vi "Rectify Image (ARGB).vi"(5 "Crop to Valid Pixels? (Default: True)":bool=TRUE, 7 "Use Fixed Point Remapping (Default: False)":bool, 8 "error in (no error)":errorcluster, 9 "ARGB Image Destination":T1, 10 "ARGB Image Source":T1, 11 "ImageRectifier":refnum<class "ImageRectifier.lvclass">) -> (0 "error out":errorcluster, 2 "ARGB Image Destination (duplicate)":T1, 3 "ImageRectifier (Duplicate)":refnum<class "ImageRectifier.lvclass">)   [LabVIEW 2020, in "image.lvlib" / "ImageRectifier.lvclass"]
uses:
  ImageRectifier.lvclass
  ARGB Image.ctl
  ImageRectifier.lvclass/ImageRectifier.ctl
  ccc224f2-fea8-4097-85c8-c2b3fe04188f.vi
  common/Module Path.vi
  <vilib>/Utility/error.llb/Error Cluster From Error Code.vi
  image.lvlib
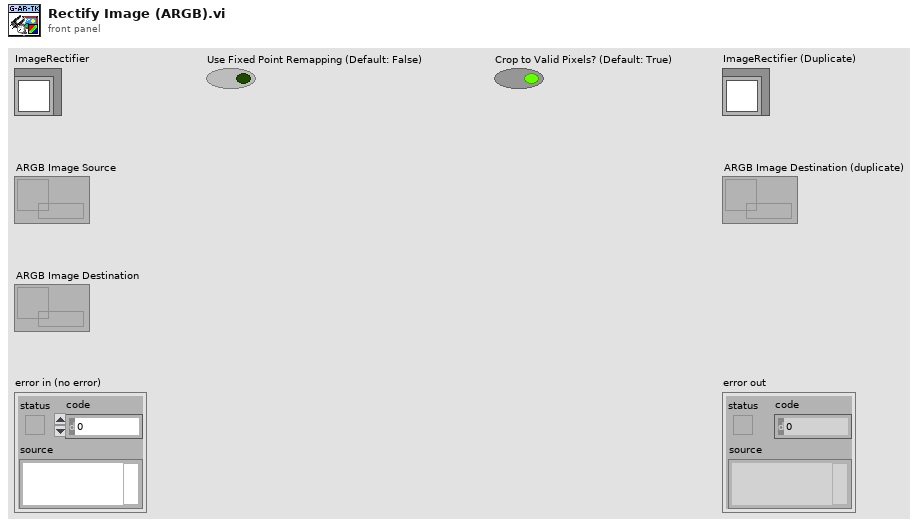
[diagram p1: front panel]
types:
  T1 = typedef "image.lvlib/ARGB Image.ctl" = refnum<data-value>
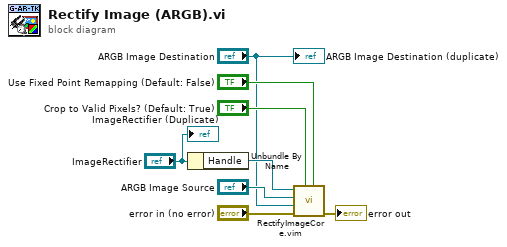
[diagram p0: block diagram]
diagram:
  n1 = Unbundle By Name("ImageRectifier") -> ("Handle"=w7:refnum<data-value>)
  n2 = call "RectifyImageCore.vim"("Use Fixed Point remapping"="Use Fixed Point Remapping (Default: False)", "Crop to Valid"="Crop to Valid Pixels? (Default: True)", "error in (no error)"="error in (no error)", "Destination Image"="ARGB Image Destination", "Source Image"="ARGB Image Source", "Handle"=w7) -> ("error out"=→"error out":errorcluster)  [unwired: 5 in]
  "ImageRectifier (Duplicate)" <- "ImageRectifier"
  "ARGB Image Destination (duplicate)" <- "ARGB Image Destination"
